vi "Graph under Cursor (SubVI).vi"(6 "AOIThreshold":dbl, 8 "error in (no error)":errorcluster, 9 "Detail Graph":refnum<vi>, 10 "Intensity Graph":refnum<vi>, 11 "Intensity Image":u16[][](array[numeric])) -> (0 "error out":errorcluster, 3 "Intensity under Cursor":u16[][](array[numeric]))   [LabVIEW 2023, in "CX Labview Wrapper.lvlib"]
uses:
  CX Labview Wrapper.lvlib
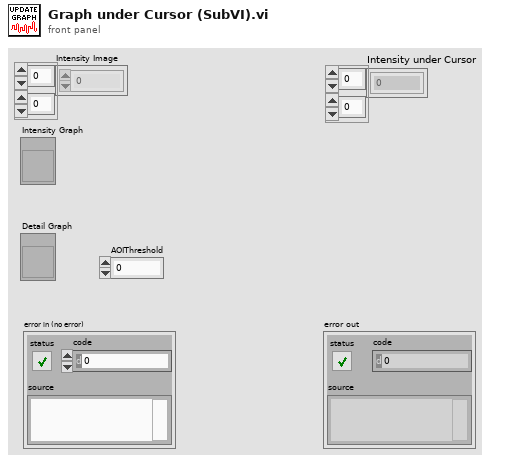
[diagram p1: front panel]
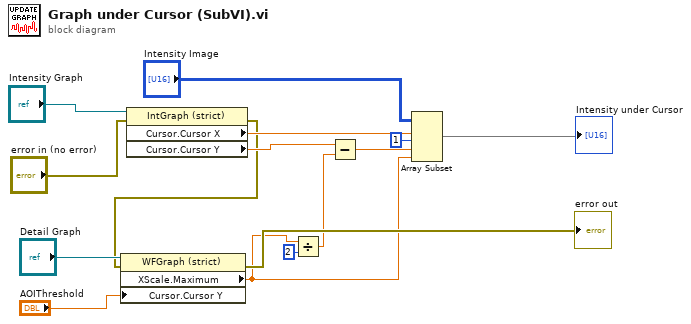
[diagram p0: block diagram]
diagram:
  n1 = property on="Property Node" class="IntGraph (strict)"(reference="Intensity Graph", error in="error in (no error)") -> (error out=w3:errorcluster, "Cursor.Cursor X"=w12:dbl, "Cursor.Cursor Y"=w14:dbl)  [unwired: 1 out]
  n2 = property on="Property Node" class="WFGraph (strict)"(reference="Detail Graph", error in=w3, "Cursor.Cursor Y"="AOIThreshold") -> (error out=→"error out":errorcluster, "XScale.Maximum"=w2:dbl)  [unwired: 1 out]
  n3 = Divide(x=w2, y=u32 2) -> (x/y=w9:dbl)
  n4 = Subtract(x=w14, y=w9) -> (x-y=w15:dbl)
  n5 = Array Subset(array="Intensity Image", index (row)=w12, length (row)=1 ("length"), index (col)=w15, length (col)=w2) -> (→"Intensity under Cursor":u16[][])
